vi "HandleItemActivation.vi"(8 "error in (no error)":errorcluster, 11 "RunVI in":refnum<class "RunVI.lvclass">) -> (0 "error out":errorcluster, 3 "RunVI out":refnum<class "RunVI.lvclass">)   [LabVIEW 2009, in "NavScreen.lvlib" / "RunVI.lvclass"]
uses:
  RunVI.lvclass
  RunVI.lvclass/RunVI.ctl
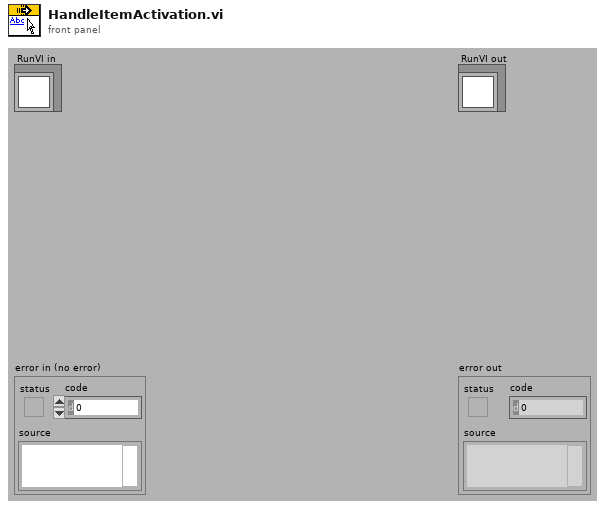
[diagram p1: front panel]
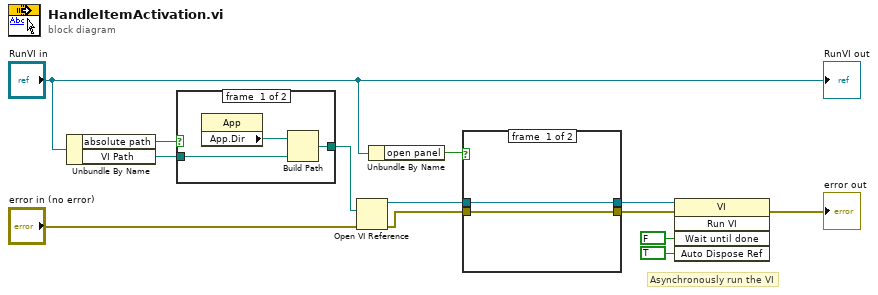
[diagram p0: block diagram]
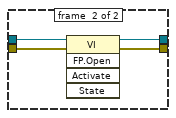
[diagram p2: hidden frame]
diagram:
  # "Asynchronously run the VI"
  n1 = Unbundle By Name("RunVI in") -> ("absolute path"=w7:bool, "VI Path"=w9:path)
  n2 = case shown="False" w7 {
    tunnel: w9 -> [w15 w17]
    tunnel: [w14 w17] -> w8
    frame #0 {
      n3 = property class="App"() -> ("App.Dir"=w16:path)  [unwired: 2 in, 2 out]
      n4 = Build Path(base path=w16, name or relative path=w15) -> (appended path=w14:path)
    }
    frame #1 {
    }
  }
  n5 = Open VI Reference(vi path=w8, error in (no error)="error in (no error)") -> (vi reference=w6:refnum<vi>, error out=w4:errorcluster)  [unwired: 4 in]
  n6 = Unbundle By Name("RunVI in") -> ("open panel"=w1:bool)
  n7 = case shown="True" w1 {
    tunnel: w6 -> [w19 w23]
    tunnel: [w19 w22] -> w5
    tunnel: w4 -> [w18 w21]
    tunnel: [w18 w20] -> w3
    frame #0 {
    }
    frame #1 {
      n8 = invoke class="VI" method="FP.Open"(reference=w23, error in=w21) -> (reference out=w22:refnum<vi>, error out=w20:errorcluster)  [unwired: 3 in, 3 out]
    }
  }
  n9 = invoke class="VI" method="Run VI"(reference=w5, error in=w3, "Wait until done"=FALSE ("Wait Until Done"), "Auto Dispose Ref"=TRUE ("Auto Dispose Reference")) -> (error out=→"error out":errorcluster)  [unwired: 1 in, 4 out]
  "RunVI out" <- "RunVI in"
